vi "macro_Rotation3d_RollPitchYaw_Deg.vi"   [LabVIEW 2019, in "Trajectory_Library.lvlib"]
uses:
  Trajectory_Library.lvlib
  Conv_Deg_Radians.vi
  VI/Quaternion_New.vi
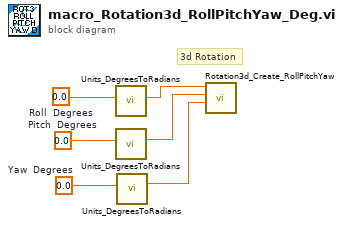
[diagram p0: block diagram]
diagram:
  w6 = 0.0  # Roll  Degrees
  w5 = 0.0  # Pitch  Degrees
  w4 = 0.0  # Yaw  Degrees
  # "3d Rotation"
  n1 = call "Units_DegreesToRadians.vi"("Degrees"=w6) -> ("Radians"=w3:dbl)  [unwired: 10 in]
  n2 = call "Units_DegreesToRadians.vi"("Degrees"=w5) -> ("Radians"=w2:dbl)  [unwired: 10 in]
  n3 = call "Units_DegreesToRadians.vi"("Degrees"=w4) -> ("Radians"=w1:dbl)  [unwired: 10 in]
  n4 = call "Rotation3d_Create_RollPitchYaw.vi"("Yaw"=w1, "Pitch"=w2, "Roll"=w3) -> ()  [unwired: 8 in, 1 out]
